vi "Align N Waveforms (single shot).vi"(4 "interpolation":bool=TRUE, 5 "exported interval":u16(ring) items=["common", "global"], 6 "FIR filter specifications":T1={"alias rejection (dB)"=120.0, "normalized bandwidth"=0.4536} {"normalized bandwidth" format="%.4f"; "alias rejection (dB)" format="%.2f"}, 7 "open interval? (T)":bool=TRUE, 8 "error in (no error)":errorcluster, 9 "interpolation mode":u16(ring)=1 items=["coerce", "linear", "spline", "FIR filter"], 11 "waveforms in":waveform(dbl)[](array[waveform])) -> (0 "error out":errorcluster, 3 "aligned waveforms out":waveform(dbl)[](array[waveform]))   [LabVIEW 2020, in "NI_MAPro.lvlib"]
doc: "Performs element-wise alignment of two waveforms and returns the aligned waveforms. The data types you wire to the waveform inputs determine the polymorphic instance to use."
uses:
  NI_MAPro.lvlib
panel:
  in  "Waveform":waveform(dbl)={"t0"=timestamp(0 s since 1904-01-01), "dt"=0.0, "Y"=[]}
  # "open"
  # "closed"
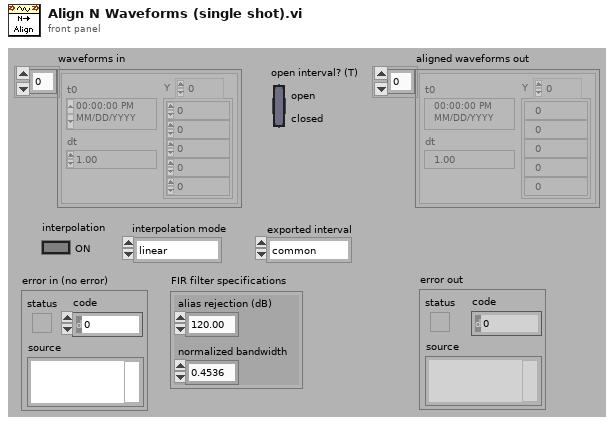
[diagram p1: front panel]
types:
  T1 = cluster{"alias rejection (dB)":dbl, "normalized bandwidth":dbl}
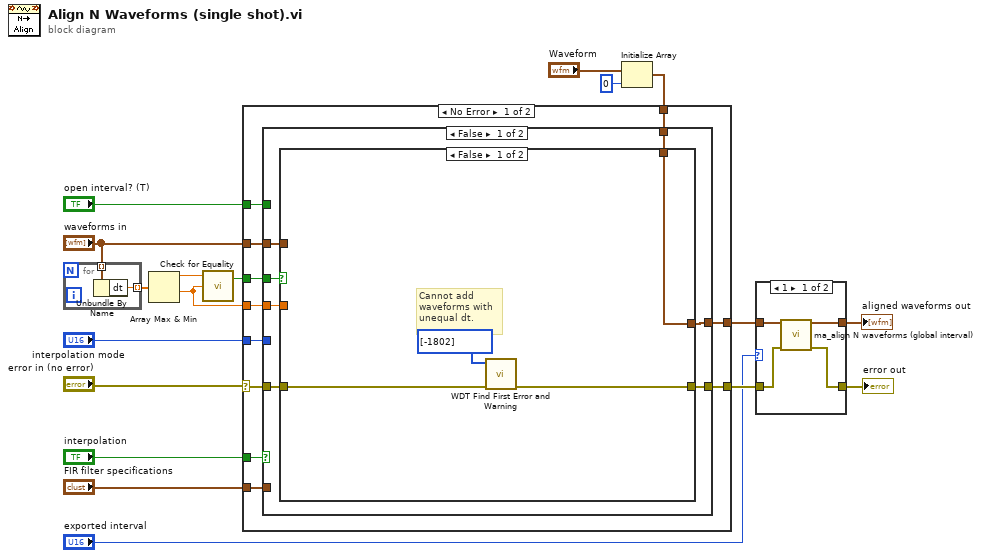
[diagram p0: block diagram]
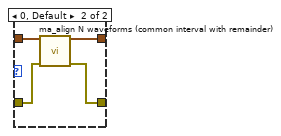
[diagram p2: hidden frame]
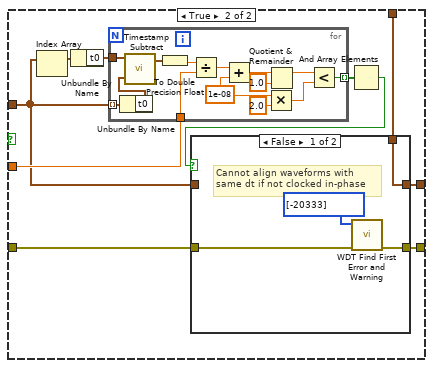
[diagram p3: hidden frame]
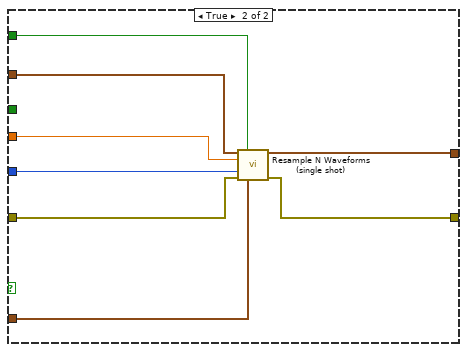
[diagram p5: hidden frame]
diagram:
  n1 = for {
    tunnel: "waveforms in" -> [w20] mode=indexing
    tunnel: [w19] -> w18 mode=indexing
    n2 = Unbundle By Name(w20) -> ("dt"=w19:dbl)
  }
  n3 = Array Max & Min(array=w18) -> (max value=w3:dbl, min value=w2:dbl)  [unwired: 2 out]
  n4 = call "Check for Equality.vi"("n2"=w2, "n1"=w3) -> ("equal?"=w1:bool)  [unwired: 1 in, 1 out]
  n5 = Initialize Array("Waveform", 0 ("dimension size")) -> (w6:waveform(dbl)[])
  n6 = case shown="No Error" "error in (no error)" {
    selector: "error in (no error)" -> [w30 w82]
    tunnel: [w29 w82] -> w14
    tunnel: w6 -> [w31 w81]
    tunnel: "interpolation mode" -> [w27 _]
    tunnel: [w28 w81] -> w15
    tunnel: "interpolation" -> [w26 _]
    tunnel: "open interval? (T)" -> [w25 _]
    tunnel: "FIR filter specifications" -> [w24 _]
    tunnel: w2 -> [w23 _]
    tunnel: "waveforms in" -> [w22 _]
    tunnel: w1 -> [w21 _]
    frame No Error {
      n7 = case shown="False" w26 {
        tunnel: w31 -> [w38 _]
        tunnel: w30 -> [w37 w79]
        tunnel: [w36 w80] -> w29
        tunnel: [w35 w75] -> w28
        tunnel: w27 -> [_ w74]
        tunnel: w25 -> [_ w78]
        tunnel: w24 -> [_ w73]
        tunnel: w23 -> [w33 w77]
        tunnel: w22 -> [w32 w76]
        tunnel: w21 -> [w34 _]
        frame False {
          n8 = case shown="False" w34 {
            tunnel: w38 -> [w39 w50]
            tunnel: w37 -> [w42 w52]
            tunnel: [w41 w51] -> w36
            tunnel: [w39 w49] -> w35
            tunnel: w33 -> [_ w48]
            tunnel: w32 -> [_ w44]
            frame False {
              # "Cannot add\nwaveforms with\nunequal dt."
              n9 = call "WDT Find First Error and Warning.vi"("error in (no error)"=w42, "Error Codes"=i32[] [-1802]) -> ("error out"=w41:errorcluster)  [unwired: 4 in, 1 out]
            }
            frame True {
              n10 = Index Array(array=w44) -> (element=w47:waveform(dbl))  [unwired: 1 in]
              n11 = Unbundle By Name(w47) -> ("t0"=w43:timestamp)
              n12 = for {
                tunnel: w43 -> [w56]
                tunnel: w48 -> [w60]
                tunnel: [w64] -> w46 mode=indexing
                tunnel: w44 -> [w59] mode=indexing
                w57 = 1e-08
                n13 = Unbundle By Name(w59) -> ("t0"=w55:timestamp)
                n14 = call "Timestamp Subtract.vi"("y"=w55, "x"=w56) -> ("x - y"=w54:timestamp)
                n15 = To Double Precision Float(number=w54) -> (double precision float=w53:dbl)
                n16 = Divide(x=w53, y=w60) -> (x/y=w58:dbl)
                n17 = Add(x=w58, y=w57) -> (x+y=w63:dbl)
                n18 = Multiply(x=w57, y=2.0) -> (x*y=w61:dbl)
                n19 = Quotient & Remainder(x=w63, y=1.0) -> (x-y*floor(x/y)=w65:dbl)  [unwired: 1 out]
                n20 = Less?(x=w65, y=w61) -> (x < y?=w64:bool)
              }
              n21 = And Array Elements(Boolean array=w46) -> (logical AND=w45:bool)
              n22 = case shown="False" w45 {
                tunnel: [w68 w71] -> w51
                tunnel: w52 -> [w67 w71]
                tunnel: w50 -> [w70 _]
                tunnel: w44 -> [_ w72]
                tunnel: [w70 w72] -> w49
                frame False {
                  # "Cannot align waveforms with\nsame dt if not clocked in-phase"
                  n23 = call "WDT Find First Error and Warning.vi"("error in (no error)"=w67, "Error Codes"=i32[] [-20333]) -> ("error out"=w68:errorcluster)  [unwired: 4 in, 1 out]
                }
                frame True {
                }
              }
            }
          }
        }
        frame True {
          n24 = call "Resample N Waveforms (single shot).vi"("waveforms in"=w76, "open interval? (F)"=w78, "dt"=w77, "interpolation mode"=w74, "error in (no error)"=w79, "FIR filter specifications"=w73) -> ("resampled waveforms out"=w75:waveform(dbl)[], "error out"=w80:errorcluster)  [unwired: 6 in, 2 out]
        }
      }
    }
    frame Error {
      # "An empty waveform is \nwritten out"
      # "Incoming Error"
    }
  }
  n25 = case shown="1" "exported interval" {
    tunnel: w15 -> [w84 w87]
    tunnel: [w86 w90] -> w13
    tunnel: w14 -> [w85 w89]
    tunnel: [w83 w88] -> w5
    frame 1 {
      n26 = call "ma_align N waveforms (global interval).vi"("waveforms in"=w84, "error in"=w85) -> ("waveforms out"=w83:waveform(dbl)[], "error out"=w86:errorcluster)  [unwired: 12 in]
    }
    frame 0, Default {
      n27 = call "ma_align N waveforms (common interval with remainder).vi"("waveforms in"=w87, "error in"=w89) -> ("intersecting waveforms out"=w88:waveform(dbl)[], "error out"=w90:errorcluster)  [unwired: 11 in, 1 out]
    }
  }
  "error out" <- w13
  "aligned waveforms out" <- w5
